vi "Autonomous.vi"   [LabVIEW 2015]
doc: "This VI starts when autonomous period begins, and will automatically be terminated when it ends. You can carry out timed or sensor driven operations directly to I/O or to subsystems without needing to return to the caller."
uses:
  <vilib>/Rock Robotics/Network Tables/NT Read String.vi
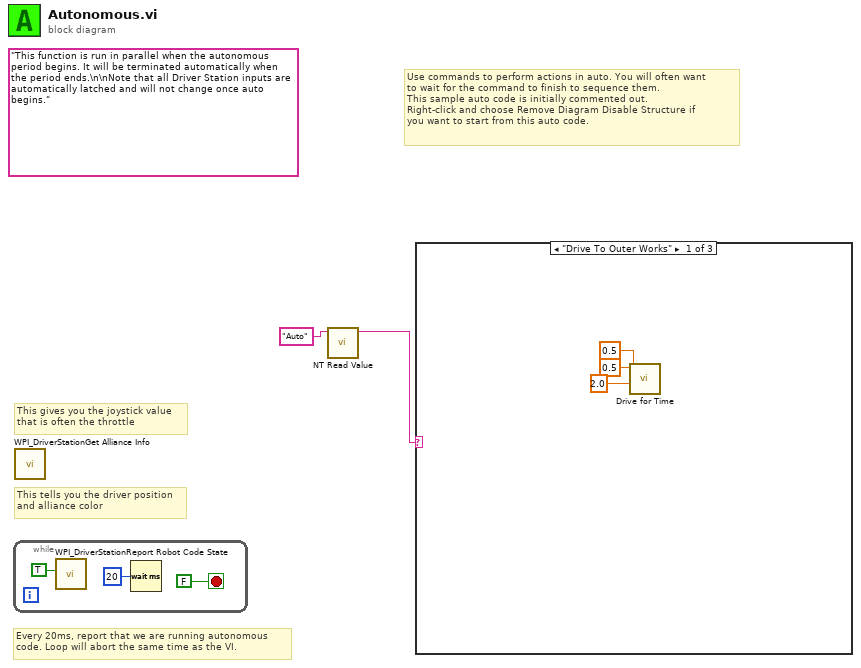
[diagram p0: block diagram]
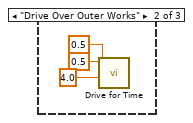
[diagram p2: hidden frame]
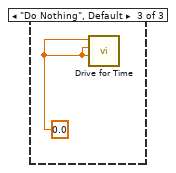
[diagram p3: hidden frame]
diagram:
  (unwired) "This function is run in parallel when the autonomous period begins. It will be terminated automatically when the period ends.\n\nNote that all Driver Station inputs are automatically latched and will not change once auto begins."
  # "Every 20ms, report that we are running autonomous\ncode. Loop will abort the same time as the VI."
  # "This gives you the joystick value\nthat is often the throttle"
  # "Use commands to perform actions in auto. You will often want\nto wait for the command to finish to sequence them.\nThis sample auto code is initially commented out. \nRight-click and choose Remove Diagram Disable Structure if\nyou want to start from this auto code."
  # "This tells you the driver position\nand alliance color"
  n1 = while {
    stop <- FALSE stop-if-true
    n2 = call <vilib>:"WPI_DriverStationReport Robot Code State.vi"("Autonomous"=TRUE) -> ()  [unwired: 10 in, 1 out]
    n3 = Wait (ms)(milliseconds to wait=u32 20) -> ()  [unwired: 1 out]
  }
  n4 = call <vilib>:"WPI_DriverStationGet Alliance Info.vi"() -> ()  [unwired: 12 out]
  n5 = call-poly <vilib>:"NT Read Value.vi"("Name"="Auto") -> ("String"=w1:string)  [unwired: 9 in, 1 out]
  n6 = case shown="\"Drive To Outer Works\"" w1 {
    frame "Drive To Outer Works" {
      n7 = call "Drive for Time.vi"("Seconds"=2.0, "Right Speed"=0.5, "Left Speed"=0.5) -> ()  [unwired: 7 in, 2 out]
    }
    frame "Drive Over Outer Works" {
      n8 = call "Drive for Time.vi"("Seconds"=4.0, "Right Speed"=0.5, "Left Speed"=0.5) -> ()  [unwired: 7 in, 2 out]
    }
    frame "Do Nothing", Default {
      w12 = 0.0
      n9 = call "Drive for Time.vi"("Seconds"=w12, "Right Speed"=w12, "Left Speed"=w12) -> ()  [unwired: 7 in, 2 out]
    }
  }
